vi "Database_Create.vi"(8 "error in (no error)":errorcluster) -> (0 "error out":errorcluster)   [LabVIEW 2013, in "Medimatic.lvlib"]
uses:
  Medimatic.lvlib
  <userlib>/LVT/SQLite/Core/Tables/SQLite_Create Table.vi
  Globals/DataPathGlobalVariable.vi
  <userlib>/_OpenG.lib/file/file.llb/File Exists - Scalar__ogtk.vi
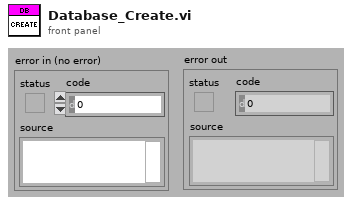
[diagram p1: front panel]
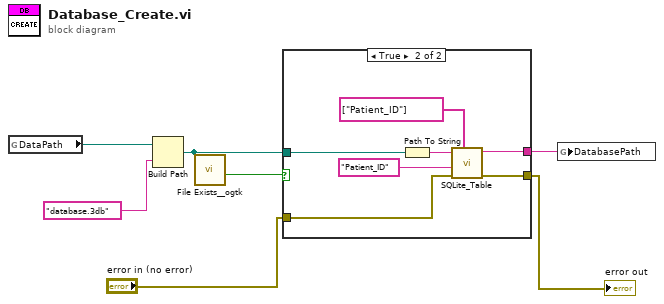
[diagram p0: block diagram]
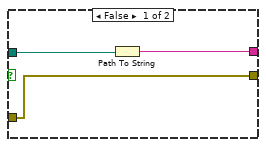
[diagram p2: hidden frame]
diagram:
  n1 = global read "DataPathGlobalVariable.vi" "DataPath"() -> (w6:path)
  n2 = Build Path(base path=w6, name or relative path="database.3db") -> (appended path=w3:path)
  n3 = call-poly <userlib>:"File Exists__ogtk.vi"("file path"=w3) -> ("exists"=w4:bool)  [unwired: 6 in, 1 out]
  n4 = case shown="True" w4 {
    tunnel: w3 -> [w10 w15]
    tunnel: [w9 w13] -> w5
    tunnel: "error in (no error)" -> [w8 w12]
    tunnel: [w8 w11] -> w1
    frame False {
      n5 = Path To String(path=w10) -> (string=w9:string)
    }
    frame True {
      n6 = Path To String(path=w15) -> (string=w14:string)
      n7 = call-poly <userlib>:"SQLite_Table.vi"("DB Path"=w14, "Table Name"="Patient_ID", "error in (no error)"=w12, "Columns"=string[] ["Patient_ID"]) -> ("DB Path Out"=w13:string, "error out"=w11:errorcluster)  [unwired: 4 in, 1 out]
    }
  }
  "error out" <- w1
  n8 = global write "DataPathGlobalVariable.vi" "DatabasePath"(w5) -> ()
